vi "fly.vi"(8 "error in (no error)":errorcluster, 11 "FlyBehavior in":refnum<class "FlyBehavior.lvclass">) -> (0 "error out":errorcluster, 2 "String":string, 3 "FlyBehavior out":refnum<class "FlyBehavior.lvclass">)   [LabVIEW 2013, in "FlyBehavior.lvclass"]
uses:
  FlyBehavior.lvclass
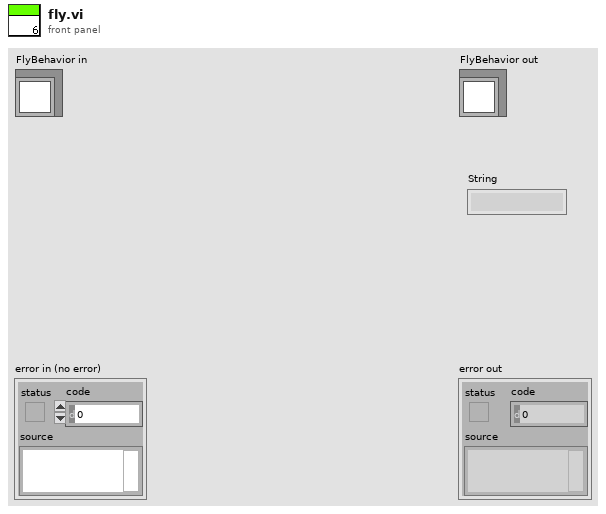
[diagram p1: front panel]
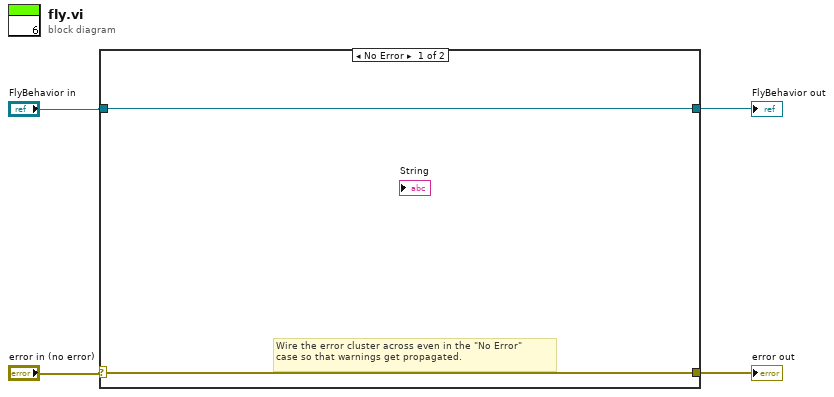
[diagram p0: block diagram]
diagram:
  n1 = case shown="No Error" "error in (no error)" {
    selector: "error in (no error)" -> [w5 w8]
    tunnel: [w5 w8] -> w2
    tunnel: [w6 w7] -> w3
    tunnel: "FlyBehavior in" -> [w6 w7]
    frame No Error {
      # "Wire the error cluster across even in the \"No Error\"\ncase so that warnings get propagated."
    }
    frame Error {
    }
  }
  "error out" <- w2
  "FlyBehavior out" <- w3
